vi "Periodic Tasks.vi"(8 "error in":errorcluster) -> ()   [LabVIEW 2015]
doc: "This VI runs in parallel to other tasks. It can contain as many user-defined periodic loops as you need. These can carry out PID or other sorts of timed response."
uses:
  <vilib>/Rock Robotics/WPI/Utilities/WPI_GetSetVariantRefNum.vi
  <vilib>/Rock Robotics/Network Tables/NT Write Number.vi
  <vilib>/Rock Robotics/Network Tables/NT Write Boolean.vi
  <vilib>/Rock Robotics/Network Tables/NT Write Numeric Array.vi
  <vilib>/Rock Robotics/Network Tables/NT Write Boolean Array.vi
  Robot Global Data.vi
  navX Library v2/navX Library v2.lvlib
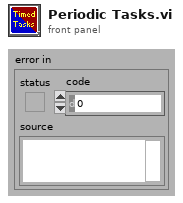
[diagram p1: front panel]
types:
  T1 = typedef "navX Library v2.lvlib/Z900_navX_DeviceTypeDef.ctl" = cluster{"Interface":cluster{"Protocol":T2, "Update Rate (4Hz-60Hz)":u8, "navX Open TypeDef":variant}, "Notify Packet":refnum<notifier>, "Loop VI Refnum":refnum<vi>, "Ready to Close Occurrence Refnum":refnum<k4>}
  T2 = typedef "navX Library v2.lvlib/Z900_navX_ProtocolTypeDef.ctl" = enum16{"SERIAL", "I2C", "SPI"}
  T3 = typedef "WPI_JoystickDevRef.ctl" = cluster{"Device":T4}
  T4 = typedef "WPI_JoystickDeviceEnum.ctl" = enum16{"USB 0", "USB 1", "USB 2", "USB 3", "USB 4", "USB 5"}
  T5 = cluster{"Yaw":dbl, "Roll":dbl, "Pitch":dbl, "Heading":dbl, "Fused Heading":dbl}
  T6 = typedef "WPI_EncoderDevRef.ctl" = cluster{"DevStatus":errorcluster, "EncoderIndex":T7, "CounterIndex":T8, "DistancePerCount":dbl, "Decoding Type":T9}
  T7 = typedef "FPGA_EncoderIdx.ctl" = enum8{"Enc 0", "Enc 1", "Enc 2", "Enc 3", "Enc 4", "Enc 5", "Enc 6", "Enc 7", "Invalid"}
  T8 = typedef "FPGA_CounterCtrSystemIndex.ctl" = enum8{"Ctr 0", "Ctr 1", "Ctr 2", "Ctr 3", "Ctr 4", "Ctr 5", "Ctr 6", "Ctr 7", "Invalid"}
  T9 = typedef "WPI_EncoderType.ctl" = enum16{"1x", "2x", "4x"}
  T10 = typedef "WPI_CompressorDevRef.ctl" = cluster{"DevStatus":errorcluster, "Pneumatics Control Module":u8}
  T11 = typedef "WPI_DriverStationRobotMode2.ctl" = enum16{"Autonomous Disabled", "Autonomous Enabled", "Teleop Disabled", "Teleop Enabled", "Disconnected", "Finish", "Test Disabled", "Test Enabled", "Emergency Stopped"}
  T12 = cluster{"POVs[0]":i16, "POVs[1]":i16, "POVs[2]":i16, "POVs[3]":i16, "POVs[4]":i16, "POVs[5]":i16, "POVs[6]":i16, "POVs[7]":i16, "POVs[8]":i16}
  T13 = cluster{"Buttons[0]":bool, "Buttons[1]":bool, "Buttons[2]":bool, "Buttons[3]":bool, "Buttons[4]":bool, "Buttons[5]":bool, "Buttons[6]":bool, "Buttons[7]":bool, "Buttons[8]":bool}
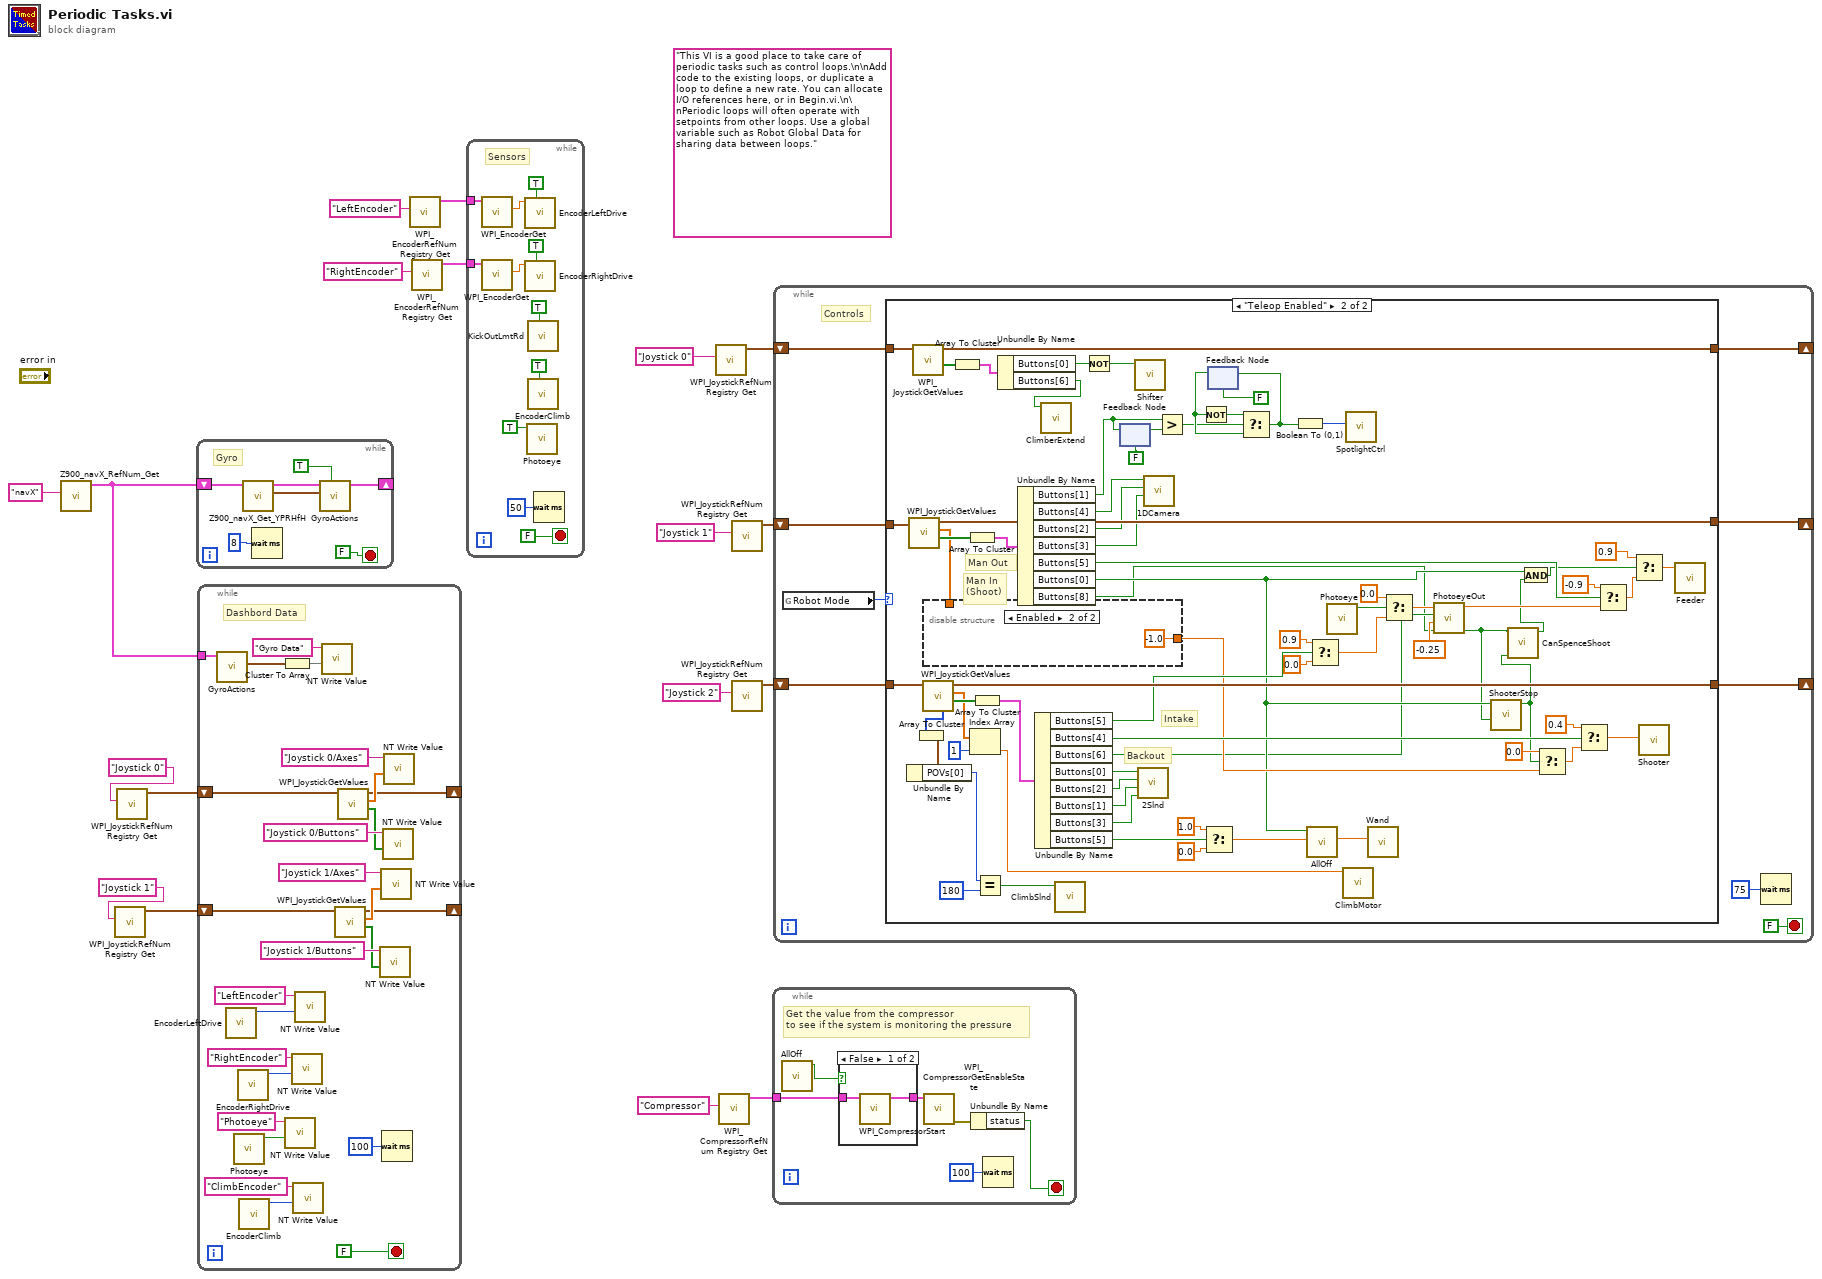
[diagram p0: block diagram]
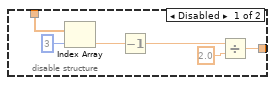
[diagram p3: hidden frame]
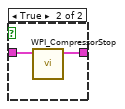
[diagram p4: hidden frame]
diagram:
  (unwired) "This VI is a good place to take care of periodic tasks such as control loops.\n\nAdd code to the existing loops, or duplicate a loop to define a new rate. You can allocate I/O references here, or in Begin.vi.\n\nPeriodic loops will often operate with setpoints from other loops. Use a global variable such as Robot Global Data for sharing data between loops."
  n1 = call "Z900_navX_RefNum_Get.vi"("refnum name"="navX") -> ("navX Device"=w17:T1)  [unwired: 9 in, 1 out]
  n2 = call <vilib>:"WPI_JoystickRefNum Registry Get.vi"("refnum name"="Joystick 1") -> ("JoystickDevRef"=w7:T3)  [unwired: 1 in, 9 out]
  n3 = call <vilib>:"WPI_JoystickRefNum Registry Get.vi"("refnum name"="Joystick 0") -> ("JoystickDevRef"=w9:T3)  [unwired: 1 in, 9 out]
  n4 = while {
    shift-right: [w19] -> _
    shift-left: w17 -> [w23]
    stop <- FALSE stop-if-true
    # "Gyro"
    n5 = call "Z900_navX_Get_YPRHfH.vi"("navX Device"=w23) -> ("YRPHfH"=w20:T5, "navX Device"=w21:T1)  [unwired: 7 in, 2 out]
    n6 = Wait (ms)(milliseconds to wait=u32 8) -> ()  [unwired: 1 out]
    n7 = call "GyroActions.vi"("Update"=TRUE, "YRPHfH_in"=w20, "navX Device"=w21) -> ("navX Device"=w19:T1)  [unwired: 4 in, 4 out]
  }
  n8 = while {
    tunnel: w17 -> [w46]
    shift-right: [w31] -> _
    shift-left: w7 -> [w33]
    shift-right: [w32] -> _
    shift-left: w9 -> [w34]
    stop <- FALSE stop-if-true
    # "Dashbord Data"
    n9 = call "GyroActions.vi"("navX Device"=w46) -> ("YRPHfH_out"=w47:T5)  [unwired: 6 in, 4 out]
    n10 = call "EncoderLeftDrive.vi"() -> ("Position_out"=w38:i32)  [unwired: 11 in]
    n11 = call "Photoeye.vi"() -> ("BeamBroken?"=w28:bool)  [unwired: 11 in]
    n12 = call "EncoderRightDrive.vi"() -> ("Position_out"=w37:i32)  [unwired: 11 in]
    n13 = call "EncoderClimb.vi"() -> ("Position_out"=w26:i32)  [unwired: 11 in]
    n14 = Cluster To Array(cluster=w47) -> (array=w51:dbl[])
    n15 = call-poly <vilib>:"NT Write Value.vi"("Boolean"=w28, "Name"="Photoeye") -> ()  [unwired: 9 in, 1 out]
    n16 = call-poly <vilib>:"NT Write Value.vi"("Numeric"=w37, "Name"="RightEncoder") -> ()  [unwired: 9 in, 1 out]
    n17 = call-poly <vilib>:"NT Write Value.vi"("Numeric"=w26, "Name"="ClimbEncoder") -> ()  [unwired: 9 in, 1 out]
    n18 = call-poly <vilib>:"NT Write Value.vi"("Numeric"=w38, "Name"="LeftEncoder") -> ()  [unwired: 9 in, 1 out]
    n19 = call-poly <vilib>:"NT Write Value.vi"("Numeric Array"=w51, "Name"="Gyro Data") -> ()  [unwired: 9 in, 1 out]
    n20 = call <vilib>:"WPI_JoystickGetValues.vi"("JoystickDevRef"=w33) -> ("Buttons"=w30:bool[], "Axes"=w39:dbl[], "JoystickDevRef"=w31:T3)  [unwired: 6 in, 2 out]
    n21 = call <vilib>:"WPI_JoystickGetValues.vi"("JoystickDevRef"=w34) -> ("Buttons"=w43:bool[], "Axes"=w42:dbl[], "JoystickDevRef"=w32:T3)  [unwired: 6 in, 2 out]
    n22 = call-poly <vilib>:"NT Write Value.vi"("Boolean Array"=w30, "Name"="Joystick 1/Buttons") -> ()  [unwired: 9 in, 1 out]
    n23 = call-poly <vilib>:"NT Write Value.vi"("Numeric Array"=w39, "Name"="Joystick 1/Axes") -> ()  [unwired: 9 in, 1 out]
    n24 = Wait (ms)(milliseconds to wait=u32 100) -> ()  [unwired: 1 out]
    n25 = call-poly <vilib>:"NT Write Value.vi"("Boolean Array"=w43, "Name"="Joystick 0/Buttons") -> ()  [unwired: 9 in, 1 out]
    n26 = call-poly <vilib>:"NT Write Value.vi"("Numeric Array"=w42, "Name"="Joystick 0/Axes") -> ()  [unwired: 9 in, 1 out]
  }
  n27 = call <vilib>:"WPI_EncoderRefNum Registry Get.vi"("refnum name"="LeftEncoder") -> ("EncoderDevRef"=w15:T6)  [unwired: 9 in, 1 out]
  n28 = call <vilib>:"WPI_EncoderRefNum Registry Get.vi"("refnum name"="RightEncoder") -> ("EncoderDevRef"=w14:T6)  [unwired: 9 in, 1 out]
  n29 = while {
    tunnel: w15 -> [w60]
    tunnel: w14 -> [w58]
    stop <- FALSE stop-if-true
    # "Sensors"
    n30 = call <vilib>:"WPI_EncoderGet.vi"("EncoderDevRef"=w60) -> ("Distance"=w59:dbl)  [unwired: 5 in, 5 out]
    n31 = call <vilib>:"WPI_EncoderGet.vi"("EncoderDevRef"=w58) -> ("Distance"=w56:dbl)  [unwired: 5 in, 5 out]
    n32 = call "EncoderLeftDrive.vi"("Update"=TRUE, "Position_in"=w59) -> ()  [unwired: 9 in, 1 out]
    n33 = call "EncoderRightDrive.vi"("Update"=TRUE, "Position_in"=w56) -> ()  [unwired: 9 in, 1 out]
    n34 = call "Photoeye.vi"("Update"=TRUE) -> ()  [unwired: 10 in, 1 out]
    n35 = call "KickOutLmtRd.vi"("Update"=TRUE) -> ()  [unwired: 10 in, 1 out]
    n36 = call "EncoderClimb.vi"("Update"=TRUE) -> ()  [unwired: 10 in, 1 out]
    n37 = Wait (ms)(milliseconds to wait=u32 50) -> ()  [unwired: 1 out]
  }
  n38 = call <vilib>:"WPI_JoystickRefNum Registry Get.vi"("refnum name"="Joystick 0") -> ("JoystickDevRef"=w2:T3)  [unwired: 1 in, 9 out]
  n39 = call <vilib>:"WPI_CompressorRefNum Registry Get.vi"("refnum name"="Compressor") -> ("CompressorDevRef"=w12:T10)  [unwired: 9 in, 1 out]
  n40 = call <vilib>:"WPI_JoystickRefNum Registry Get.vi"("refnum name"="Joystick 1") -> ("JoystickDevRef"=w3:T3)  [unwired: 1 in, 9 out]
  n41 = call <vilib>:"WPI_JoystickRefNum Registry Get.vi"("refnum name"="Joystick 2") -> ("JoystickDevRef"=w1:T3)  [unwired: 1 in, 9 out]
  n42 = while {
    tunnel: w12 -> [w68]
    stop <- w66 stop-if-true
    # "Get the value from the compressor \nto see if the system is monitoring the pressure"
    n43 = call "AllOff.vi"() -> ("Compressor"=w63:bool)  [unwired: 8 in, 3 out]
    n44 = case shown="False" w63 {
      tunnel: w68 -> [w70 w72]
      tunnel: [w69 w71] -> w65
      frame False {
        n45 = call <vilib>:"WPI_CompressorStart.vi"("CompressorDevRef"=w70) -> ("CompressorDevRef"=w69:T10)  [unwired: 9 in, 1 out]
      }
      frame True {
        n46 = call <vilib>:"WPI_CompressorStop.vi"("CompressorDevRef"=w72) -> ("CompressorDevRef"=w71:T10)  [unwired: 9 in, 1 out]
      }
    }
    n47 = call <vilib>:"WPI_CompressorGetEnableState.vi"("CompressorDevRef"=w65) -> ("error out"=w64:errorcluster)  [unwired: 1 in, 9 out]
    n48 = Unbundle By Name(w64) -> ("status"=w66:bool)
    n49 = Wait (ms)(milliseconds to wait=u32 100) -> ()  [unwired: 1 out]
  }
  n50 = while {
    shift-right: [w74] -> _
    shift-left: w3 -> [w79]
    shift-right: [w75] -> _
    shift-left: w2 -> [w78]
    shift-right: [w76] -> _
    shift-left: w1 -> [w77]
    stop <- FALSE stop-if-true
    # "Controls"
    n51 = global read "Robot Global Data.vi" "Robot Mode"() -> (w73:T11)
    n52 = case shown="\"Teleop Enabled\"" w73 {
      tunnel: w79 -> [w83 w143]
      tunnel: w78 -> [w84 w142]
      tunnel: w77 -> [w82 w141]
      tunnel: [w82 w140] -> w76
      tunnel: [w84 w139] -> w75
      tunnel: [w83 w138] -> w74
      frame "Autonomous Disabled", Default {
      }
      frame "Teleop Enabled" {
        # "Backout"
        # "Intake"
        # "Man In\n(Shoot)"
        # "Man Out"
        n53 = call <vilib>:"WPI_JoystickGetValues.vi"("JoystickDevRef"=w143) -> ("Buttons"=w156:bool[], "Axes"=w154:dbl[], "JoystickDevRef"=w138:T3)  [unwired: 6 in, 2 out]
        n54 = call <vilib>:"WPI_JoystickGetValues.vi"("JoystickDevRef"=w142) -> ("Buttons"=w145:bool[], "JoystickDevRef"=w139:T3)  [unwired: 6 in, 3 out]
        n55 = call <vilib>:"WPI_JoystickGetValues.vi"("JoystickDevRef"=w141) -> ("Buttons"=w146:bool[], "Axes"=w106:dbl[], "JoystickDevRef"=w140:T3, "POVs"=w92:i16[])  [unwired: 6 in, 1 out]
        n56 = Array To Cluster(array=w92) -> (cluster=w91:T12)
        n57 = Unbundle By Name(w91) -> ("POVs[0]"=w90:i16)
        n58 = disable-structure shown="Enabled" {
          disable-tunnel: w154 -> [w162 _]
          disable-tunnel: [w157 -1.0] -> w98
          frame Disabled {
            n59 = Index Array(array=w162, index=3) -> (element=w160:dbl)
            n60 = Decrement(x=w160) -> (x-1=w159:dbl)
            n61 = Divide(x=w159, y=2.0) -> (x/y=w157:dbl)
          }
          frame Enabled {
          }
        }
        n62 = Array To Cluster(array=w145) -> (cluster=w135:T13)
        n63 = Array To Cluster(array=w156) -> (cluster=w136:T13)
        n64 = Index Array(array=w106, index=1) -> (element=w104:dbl)
        n65 = Array To Cluster(array=w146) -> (cluster=w155:T13)
        n66 = Equal?(x=w90, y=i16 180) -> (x = y?=w88:bool)
        n67 = Unbundle By Name(w135) -> ("Buttons[0]"=w102:bool, "Buttons[6]"=w87:bool)
        n68 = Unbundle By Name(w136) -> ("Buttons[1]"=w120:bool, "Buttons[4]"=w130:bool, "Buttons[2]"=w129:bool, "Buttons[3]"=w128:bool, "Buttons[5]"=w111:bool, "Buttons[0]"=w96:bool, "Buttons[8]"=w85:bool)
        n69 = Unbundle By Name(w155) -> ("Buttons[5]"=w108:bool, "Buttons[4]"=w117:bool, "Buttons[6]"=w86:bool, "Buttons[0]"=w150:bool, "Buttons[2]"=w149:bool, "Buttons[1]"=w148:bool, "Buttons[3]"=w147:bool, "Buttons[5]"=w137:bool)
        n70 = call "ClimberExtend.vi"("Button"=w87) -> ()  [unwired: 11 in]
        n71 = call "ClimbSlnd.vi"("Button"=w88) -> ()  [unwired: 11 in]
        n72 = Not(x=w102) -> (.not. x?=w101:bool)
        n73 = feedback-in #1(w120) -> ()
        n74 = feedback #1(FALSE) -> (w122:bool)
        n75 = call "Shifter.vi"("Shift"=w101) -> ()  [unwired: 11 in]
        n76 = call "2Slnd.vi"("AllUp"=w147, "AllDown"=w148, "MostUp"=w149, "MostDown"=w150) -> ()  [unwired: 8 in]
        n77 = call "1DCamera.vi"("Angle3"=w128, "Angle2"=w129, "Angle1"=w130) -> ()  [unwired: 9 in]
        n78 = Greater?(x=w120, y=w122) -> (0:w121:bool)
        n79 = Select(t=1.0, s=w137, f=0.0) -> (s? t:f=w134:dbl)
        n80 = feedback #2(FALSE) -> (w124:bool)
        n81 = Not(x=w124) -> (.not. x?=w126:bool)
        n82 = Select(t=w126, s=w121, f=w124) -> (s? t:f=w123:bool)
        n83 = feedback-in #2(w123) -> ()
        n84 = Boolean To (0,1)(Boolean=w123) -> (0, 1=w119:i16)
        n85 = call "AllOff.vi"("WandIn"=w134, "ButtonIn"=w96) -> ("WandOut"=w133:dbl)  [unwired: 6 in, 3 out]
        n86 = Select(t=0.9, s=w108, f=0.0) -> (s? t:f=w115:dbl)
        n87 = call "Photoeye.vi"() -> ("BeamBroken?"=w100:bool)  [unwired: 11 in]
        n88 = call "ClimbMotor.vi"("Power"=w104) -> ()  [unwired: 11 in]
        n89 = call "SpotlightCtrl.vi"("Direction"=w119) -> ()  [unwired: 11 in]
        n90 = call "Wand.vi"("Power"=w133) -> ()  [unwired: 11 in]
        n91 = Select(t=0.0, s=w100, f=w115) -> (s? t:f=w110:dbl)
        n92 = call "PhotoeyeOut.vi"("Hard Stop"=w85, "MotorPower"=-0.25, "Button"=w86, "MotorIn"=w110) -> ("Complete"=w94:bool, "MotorOut"=w109:dbl)  [unwired: 6 in]
        n93 = call "ShooterStop.vi"("Run"=w94, "Button"=w96) -> ("StopShooter?"=w95:bool)  [unwired: 9 in]
        n94 = call "CanSpenceShoot"("Shooter Stopped?"=w95, "Ball Out?"=w94) -> ("CanSpenceShoot?"=w93:bool)  [unwired: 9 in]
        n95 = And(x=w96, y=w93) -> (x .and. y?=w99:bool)
        n96 = Select(t=0.0 ("f"), s=w95, f=w98) -> (s? t:f=w103:dbl)
        n97 = Select(t=0.4, s=w117, f=w103) -> (s? t:f=w132:dbl)
        n98 = Select(t=-0.9, s=w111, f=w109) -> (s? t:f=w114:dbl)
        n99 = Select(t=0.9, s=w99, f=w114) -> (s? t:f=w112:dbl)
        n100 = call "Shooter.vi"("Power"=w132) -> ()  [unwired: 11 in]
        n101 = call "Feeder.vi"("Power"=w112) -> ()  [unwired: 11 in]
      }
    }
    n102 = Wait (ms)(milliseconds to wait=u32 75) -> ()  [unwired: 1 out]
  }
